vi "Thermal Chamber Controller_DQMH_Action Update Ramp Rate-with-queue-teardown.vi"(8 "error out":errorcluster, 11 "test case ID":string) -> (3 "result":bool)   [LabVIEW 2018]
doc: "The teardown VI should be executed after the VI under test in the harness VI. In this VI you can evaluate the outputs of the VI under test.\n\nSee the Help Document for more information. (<b>Help</b> > <b>IncQuery Labs</b> > <b>InstaCoverage</b> > <b>InstaCoverage Help...</b>)"
uses:
  Libraries/Thermal Chamber Response Simulator/Thermal Chamber Response Simulator.lvlib
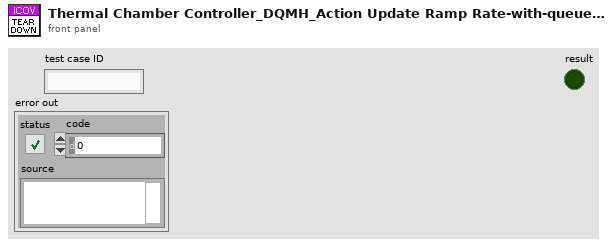
[diagram p1: front panel]
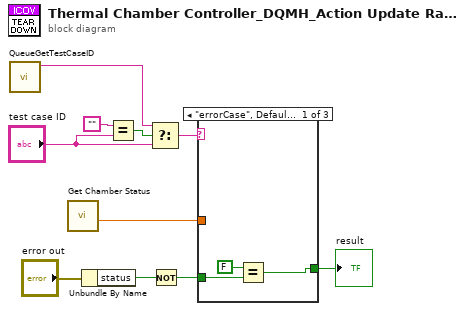
[diagram p0: block diagram]
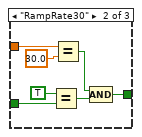
[diagram p2: hidden frame]
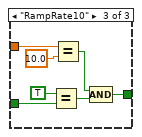
[diagram p3: hidden frame]
diagram:
  n1 = call "QueueGetTestCaseID.vi"() -> ("test case ID"=w5:string)  [unwired: 11 in]
  n2 = call "Get Chamber Status.vi"() -> ("Ramp Rate (deg C / second)"=w6:dbl)  [unwired: 6 in, 5 out]
  n3 = Unbundle By Name("error out") -> ("status"=w10:bool)
  n4 = Equal?(x="", y="test case ID") -> (x = y?=w4:bool)
  n5 = Select(t=w5, s=w4, f="test case ID") -> (s? t:f=w2:string)
  n6 = Not(x=w10) -> (.not. x?=w8:bool)
  n7 = case shown="\"errorCase\", Default" w2 {
    tunnel: w8 -> [w11 w15 w27]
    tunnel: w6 -> [_ w16 w24]
    tunnel: [w12 w14 w21] -> w7
    frame "errorCase", Default {
      n8 = Equal?(x=FALSE, y=w11) -> (x = y?=w12:bool)
    }
    frame "RampRate30" {
      n9 = Equal?(x=TRUE, y=w15) -> (x = y?=w17:bool)
      n10 = Equal?(x=w16, y=30.0) -> (x = y?=w18:bool)
      n11 = Compound Arithmetic op=AND(w18, w17) -> (w14:bool)
    }
    frame "RampRate10" {
      n12 = Equal?(x=TRUE, y=w27) -> (x = y?=w22:bool)
      n13 = Equal?(x=w24, y=10.0) -> (x = y?=w23:bool)
      n14 = Compound Arithmetic op=AND(w23, w22) -> (w21:bool)
    }
  }
  "result" <- w7
